vi "set authorizer.vi"(8 "error in (no error)":errorcluster, 9 "pUserData":u32, 10 "?":i32, 11 "para0":dbl) -> (0 "error out":errorcluster, 1 "pUserData out":u32, 2 "function return":i32, 3 "para0 out":dbl)   [LabVIEW 2020, in "sqlite3.lvlib"]
uses:
  sqlite3.lvlib
  errstr.vi
  bin/sqlite3_64.dll
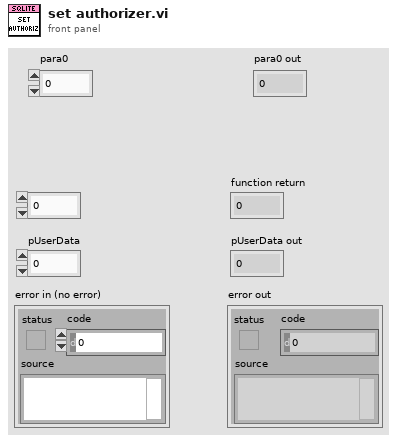
[diagram p1: front panel]
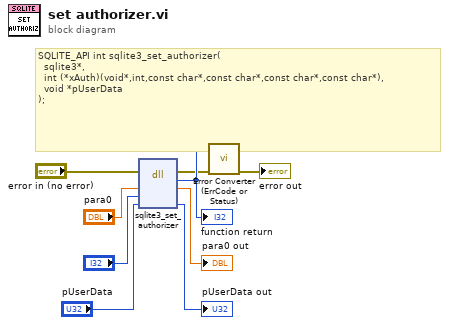
[diagram p0: block diagram]
diagram:
  # "SQLITE_API int sqlite3_set_authorizer(\n  sqlite3*,\n  int (*xAuth)(void*,int,const char*,const char*,const char*,const char*),\n  void *pUserData\n);"
  n1 = dll-call lib="D:/Project/Labview-Projects/database-configuration/externals/sqlite3/Source/bin/sqlite3_*.*" fn="sqlite3_set_authorizer"(error in="error in (no error)", "para0"="para0", "?", "pUserData"="pUserData") -> (error out=w2:errorcluster, w9:i32, "para0"=→"para0 out":dbl, "pUserData"=→"pUserData out":u32)  [unwired: 3 in, 1 out]
  "function return" <- w9
  n2 = call "Error Converter (ErrCode or Status).vi"("error in (no error)"=w2, "error code"=w9) -> ("error out"=→"error out":errorcluster)  [unwired: 9 in]
